vi "myRIO_BRig_RT_dataLC_Cue1_delayOpt_Switch_l1.vi"() -> (2 "output_Cue1_delayOpt_Switch_l1":i32)   [LabVIEW 2014]
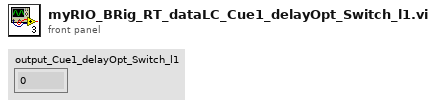
[diagram p1: front panel]
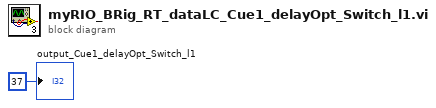
[diagram p0: block diagram]
diagram:
  "output_Cue1_delayOpt_Switch_l1" <- 37 ("output_iBlock")
